vi "Decimal to BCD.vi"(10 "size in bits":u32, 11 "decimal data in":u16) -> (3 "bcd data out":u16 format="%.0b")   [LabVIEW 2020, in "dt_encodeDecode.lvlib"]
uses:
  dt_encodeDecode.lvlib
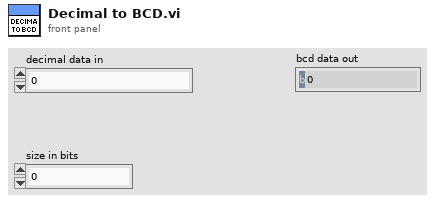
[diagram p1: front panel]
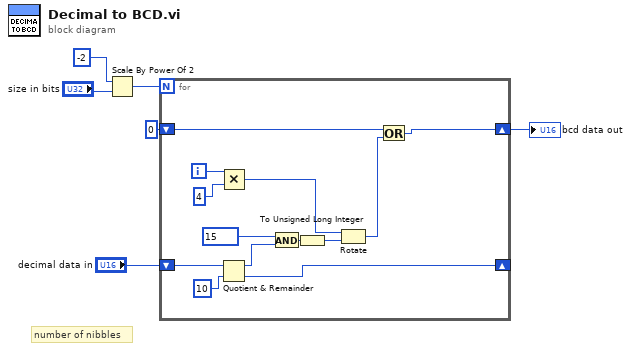
[diagram p0: block diagram]
diagram:
  # "number of nibbles"
  n1 = Scale By Power Of 2(n=-2 ("index"), x="size in bits") -> (x*2^n=w4:u32)
  n2 = for {
    N: w4 -> [_]
    shift-right: [w17] -> _
    shift-left: "decimal data in" -> [w18]
    shift-right: [w8] -> w1
    shift-left: u16 0 -> [w9]
    i -> [w14]
    n3 = Multiply(x=w14, y=4) -> (x*y=w12:i32)
    n4 = Quotient & Remainder(x=w18, y=u16 10) -> (x-y*floor(x/y)=w16:u16, floor(x/y)=w17:u16)
    n5 = And(x=u16 15 ("y"), y=w16) -> (x .and. y?=w11:u16)
    n6 = To Unsigned Long Integer(number=w11) -> (unsigned 32bit integer=w7:u32)
    n7 = Rotate(1:w7, 2:w12) -> (0:w15:u32)
    n8 = Or(x=w9, y=w15) -> (x .or. y?=w8:u32)
  }
  "bcd data out" <- w1
